vi "mes~产品出站.vi"(8 "error in (no error)":errorcluster caption="错误输入（无错误）", 11 "测试结果":string caption="测试结果:") -> (0 "error out":errorcluster caption="错误输出", 1 "ErrorMessage":string, 2 "出站成功":bool)   [LabVIEW 2020]
uses:
  Global.vi
  <vilib>/addons/_JKI.lib/Serialization/JSON/JKI JSON Serialization.lvlib
panel:
  in  "Headers":string[][](array[string])=[["Content-Type", "application/json"]]
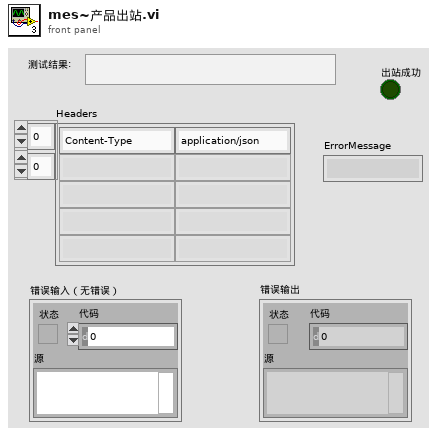
[diagram p1: front panel]
types:
  T1 = cluster{"equipmentCode":string, "productBarcode":string, "passed":i32, "ngCode":string}
  T2 = cluster{"接口地址(URL)":string, "用户登录":string, "产品进站":string, "参数采集":string, "产品出站":string, "设备状态":string, "设备编号(equipNum)":string, "站点名称(siteCode)":string, "生产类型(productType)":string, "追溯编号(traceCode)":string}
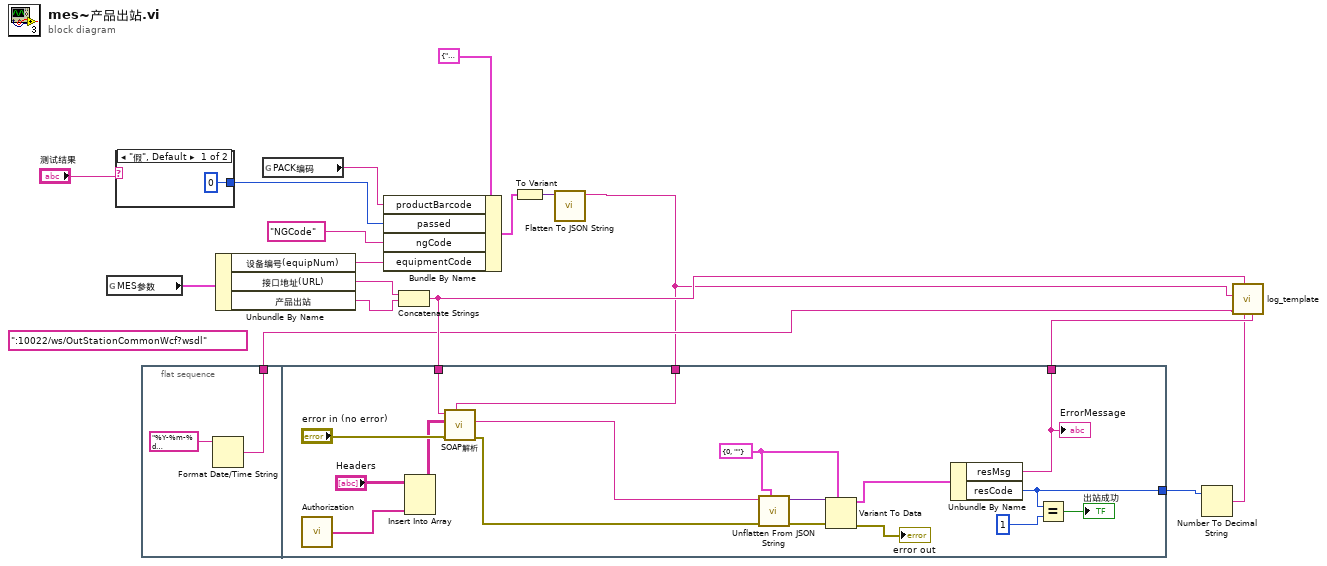
[diagram p0: block diagram]
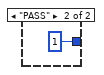
[diagram p2: hidden frame]
diagram:
  (unwired) ":10022/ws/OutStationCommonWcf?wsdl"
  n1 = global read "Global.vi" "MES参数"() -> (w15:T2)
  n2 = case shown="\"假\", Default" "测试结果" {
    tunnel: [0 1] -> w5
    frame "假", Default {
    }
    frame "PASS" {
    }
  }
  n3 = flat-sequence {
    tunnel: [w20] -> w11
    tunnel: w8 -> [w35]
    tunnel: w12 -> [w36]
    tunnel: [w34] -> w10
    tunnel: [w33] -> w3
    frame #0 {
      n4 = Format Date/Time String(time format string (%c)="%Y-%m-%d %H:%M:%S%3u-->" ("EndTime")) -> (date/time string=w20:string)  [unwired: 2 in]
    }
    frame #1 {
      w26 = cluster{"resCode":i32, "resMsg":string} {"resCode"=0, "resMsg"=""} ("用户登录ctl")
      n5 = call "Authorization.vi"() -> ("Authorization"=w32:string[])
      n6 = Insert Into Array(array="Headers", new element=w32) -> (w30:string[][])  [unwired: 2 in]
      n7 = call "SOAP解析.vi"("DATA"=w35, "错误输入（无错误）"="error in (no error)", "Headers"=w30, "URL"=w36) -> ("错误输出"=w24:errorcluster, "body"=w25:string)  [unwired: 5 in, 1 out]
      n8 = call <vilib>:"Unflatten From JSON String.vi"("Type and Defaults"=w26, "error in (no error)"=w24, "JSON String"=w25) -> ("error out"=w28:errorcluster, "Variant"=w29:variant)  [unwired: 7 in]
      n9 = Variant To Data(error in=w28, type=w26, Variant=w29) -> (data=w23:cluster{"resCode":i32, "resMsg":string}, error out=→"error out":errorcluster)
      n10 = Unbundle By Name(w23) -> ("resMsg"=w34:string, "resCode"=w33:i32)
      "ErrorMessage" <- w34
      n11 = Equal?(x=w33, y=1) -> (x = y?=→"出站成功":bool)
    }
  }
  n12 = Unbundle By Name(w15) -> ("设备编号(equipNum)"=w16:string, "接口地址(URL)"=w1:string, "产品出站"=w13:string)
  n13 = global read "Global.vi" "PACK编码"() -> (w6:string)
  n14 = Bundle By Name(cluster=T1 {"equipmentCode"="E1000121", "productBarcode"="B3332AE100531", "passed"=0, "ngCode"="N09"} ("用户登录ctl"), "productBarcode"=w6, "passed"=w5, "ngCode"="NGCode", "equipmentCode"=w16) -> (w17:T1)
  n15 = Concatenate Strings(w1, w13) -> (w12:string)
  n16 = To Variant(anything=w17) -> (Variant=w9:variant)
  n17 = call <vilib>:"Flatten To JSON String.vi"("Variant"=w9) -> ("JSON String"=w8:string)  [unwired: 9 in, 1 out]
  n18 = Number To Decimal String(number=w3) -> (decimal integer string=w2:string)  [unwired: 1 in]
  n19 = call "log_template.vi"("接收报文"=w10, "a:Success"=w2, "URL"=w12, "StartTime"=w11, "发送报文"=w8) -> ()  [unwired: 7 in]
